vi "Create From Variant.vi"(8 "error in (no error)":errorcluster, 11 "value":variant) -> (0 "error out":errorcluster, 2 "name":string, 3 "Type Definition out":refnum<class "Type Definition.lvclass">)   [LabVIEW 2020, in "PV Access.lvlib" / "PV Data.lvlib" / "Type Definition.lvclass"]
uses:
  Type Definition.lvclass
  <userlib>/_OpenG.lib/lvdata/lvdata.llb/openg_variant.lvlib
  PV Data.lvlib
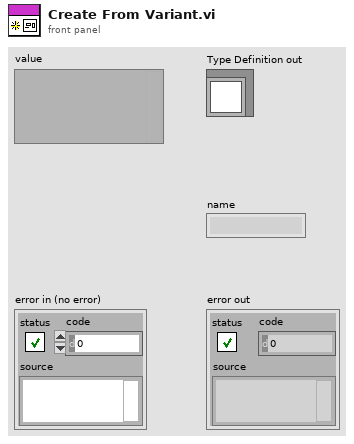
[diagram p1: front panel]
types:
  T1 = typedef "PV Access.lvlib/PV Data.lvlib/Type Code.ctl" = enum8{"Null", "Bool", "BoolA", "Int8", "Int8A", "Int16", "Int16A", "Int32", "Int32A", "Int64", "Int64A", "UInt8", "UInt8A", "UInt16", "UInt16A", "UInt32", "UInt32A", "UInt64", "UInt64A", "Float32", "Float32A", "Float64", "Float64A", "String", "StringA", "Struct", "StructA", "Union", "UnionA", "Any", "AnyA"}
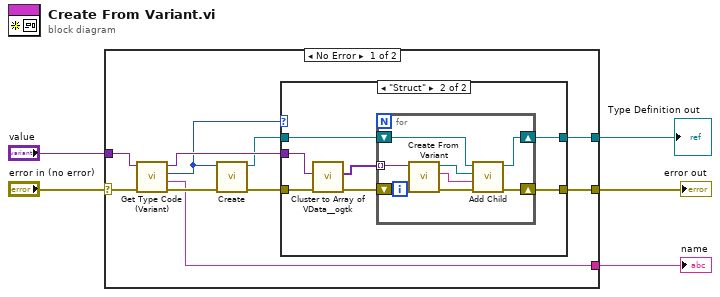
[diagram p0: block diagram]
diagram:
  n1 = case shown="No Error" "error in (no error)" {
    selector: "error in (no error)" -> [w15 w33]
    tunnel: [w9 w33] -> w4
    tunnel: [w8 _] -> w3
    tunnel: "value" -> [w14 _]
    tunnel: [w7 _] -> w1
    frame No Error {
      n2 = call "Get Type Code (Variant).vi"("error in (no error)"=w15, "value"=w14) -> ("error out"=w12:errorcluster, "name"=w7:string, "type code"=w6:T1, "value dup"=w13:variant)  [unwired: 4 in]
      n3 = call "Create.vi"("error in (no error)"=w12, "type code"=w6) -> ("error out"=w11:errorcluster, "Type Definition out"=w10:refnum<class "Type Definition.lvclass">)  [unwired: 8 in]
      n4 = case shown="\"Struct\"" w6 {
        tunnel: w13 -> [_ w24]
        tunnel: [w16 w21] -> w8
        tunnel: [w17 w20] -> w9
        tunnel: w11 -> [w17 w18]
        tunnel: w10 -> [w16 w19]
        frame Default {
        }
        frame "Struct" {
          n5 = call <userlib>:"Cluster to Array of VData__ogtk.vi"("error in (no error)"=w18, "Cluster"=w24) -> ("error out"=w23:errorcluster, "Array of VData"=w22:variant[])  [unwired: 8 in]
          n6 = for {
            shift-right: [w31] -> w20
            shift-left: w23 -> [w29]
            tunnel: w22 -> [w25] mode=indexing
            shift-right: [w30] -> w21
            shift-left: w19 -> [w32]
            n7 = call "Create From Variant.vi"("error in (no error)"=w29, "value"=w25) -> ("error out"=w28:errorcluster, "name"=w26:string, "Type Definition out"=w27:refnum<class "Type Definition.lvclass">)  [unwired: 7 in]
            n8 = call-dynamic "Add Child.vi"("error in (no error)"=w28, "name"=w26, "child"=w27, "Type Definition in"=w32) -> ("error out"=w31:errorcluster, "Type Definition out"=w30:refnum<class "Type Definition.lvclass">)  [unwired: 6 in]
          }
        }
      }
    }
    frame Error {
    }
  }
  "error out" <- w4
  "Type Definition out" <- w3
  "name" <- w1
